vi "Setup Multiple Statistics Measurement.vi"(6 "Measurements":T1[](array[typedef]), 8 "error in (no error)":errorcluster, 10 "Channels":T2, 11 "MSOX6004 in":refnum<class "MSOX6004.lvclass">) -> (0 "error out":errorcluster, 3 "MSOX6004 out":refnum<class "MSOX6004.lvclass">)   [LabVIEW 2018, in "MSOX6004.lvlib" / "MSOX6004.lvclass"]
uses:
  MSOX6004.lvclass
  PPLs/Oscilloscope/Parent/Oscilloscope.lvlibp/Custom Controls/Analog Channels.ctl
  PPLs/Oscilloscope/Parent/Oscilloscope.lvlibp/Custom Controls/Measurement.ctl
  MSOX6004.lvclass/MSOX6004.ctl
  <instrlib>/Keysight InfiniiVision/Keysight InfiniiVision.lvlib
  PPLs/Oscilloscope/Parent/Oscilloscope.lvlibp/Oscilloscope.lvclass
  C:/Projects/LabVIEW/PPLs/Oscilloscope/Parent/Oscilloscope.lvlibp/Oscilloscope.lvclass
  PPLs/Oscilloscope/Parent/Oscilloscope.lvlibp
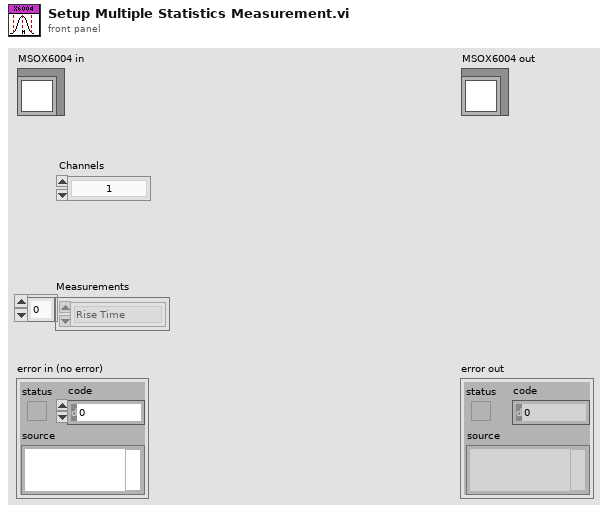
[diagram p1: front panel]
types:
  T1 = typedef "Oscilloscope.lvlibp/Measurement.ctl" = enum16{"Rise Time", "Fall Time", "Frequency", "Period", "RMS (V)", "Peak-Peak (V)", "Max (V)", "Min (V)", "High State (V)", "Low State (V)", "Average (V)", "Width (Negative)", "Width (Positive)", "Duty Cycle (Negative)", "Duty Cycle (Positive)", "Amplitude", "Cycle RMS (V)", "Cycle Avg (V)", "Overshoot", "Preshoot", "Time at Max", "Frequency Counter", "Time at Min", "Delay", "Value at Time", "Phase", "Time at Value", "Time of Edge", "Area", "Burst Width", "Falling Edge Count", "Rising Edge Count", "Falling Pulse Count", "Rising Pulse Count", "Std Dev", "Pulse Width"}
  T2 = typedef "Oscilloscope.lvlibp/Analog Channels.ctl" = enum16{"1", "2", "3", "4", "5", "6", "7", "8", "9", "10", "11", "12", "13", "14", "15", "16"}
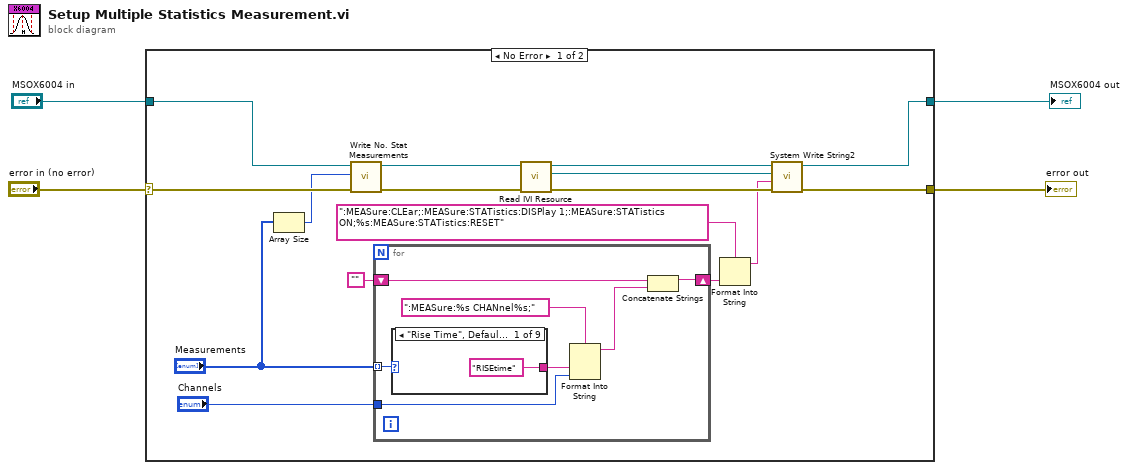
[diagram p0: block diagram]
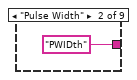
[diagram p2: hidden frame]
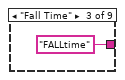
[diagram p3: hidden frame]
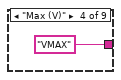
[diagram p4: hidden frame]
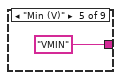
[diagram p5: hidden frame]
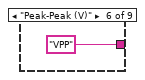
[diagram p6: hidden frame]
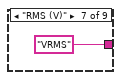
[diagram p7: hidden frame]
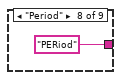
[diagram p8: hidden frame]
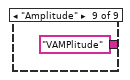
[diagram p9: hidden frame]
diagram:
  n1 = case shown="No Error" "error in (no error)" {
    selector: "error in (no error)" -> [w8 w36]
    tunnel: "MSOX6004 in" -> [w10 w37]
    tunnel: [w11 w37] -> w1
    tunnel: [w13 w36] -> w3
    frame No Error {
      n2 = Array Size(array="Measurements") -> (size(s)=w5:i32)
      n3 = call "Write No. Stat Measurements.vi"("error in (no error)"=w8, "No. Stat Measurements"=w5, "Oscilloscope in"=w10) -> ("error out"=w7:errorcluster, "Oscilloscope out"=w9:refnum<class "MSOX6004.lvclass">)  [unwired: 7 in]
      n4 = for {
        tunnel: "Measurements" -> [w26] mode=indexing
        tunnel: "Channels" -> [w24]
        shift-right: [w22] -> w17
        shift-left: "" -> [w21]
        n5 = case shown="\"Rise Time\", Default" w26 {
          tunnel: ["RISEtime" "PWIDth" "FALLtime" "VMAX" "VMIN" "VPP" "VRMS" "PERiod" "VAMPlitude"] -> w25
          frame "Rise Time", Default {
          }
          frame "Pulse Width" {
          }
          frame "Fall Time" {
          }
          frame "Max (V)" {
          }
          frame "Min (V)" {
          }
          frame "Peak-Peak (V)" {
          }
          frame "RMS (V)" {
          }
          frame "Period" {
          }
          frame "Amplitude" {
          }
        }
        n6 = Format Into String(format string=":MEASure:%s CHANnel%s;", w25, w24) -> (resulting string=w20:string)  [unwired: 2 in, 1 out]
        n7 = Concatenate Strings(w21, w20) -> (w22:string)
      }
      n8 = call "Read IVI Resource.vi"("error in (no error)"=w7, "MSOX6004 in"=w9) -> ("error out"=w15:errorcluster, "IVI Resource"=w16:refnum<k15>, "MSOX6004 out"=w11:refnum<class "MSOX6004.lvclass">)  [unwired: 7 in]
      n9 = Format Into String(format string=":MEASure:CLEar;:MEASure:STATistics:DISPlay 1;:MEASure:STATistics ON;%s:MEASure:STATistics:RESET", w17) -> (resulting string=w14:string)  [unwired: 2 in, 1 out]
      n10 = call <instrlib>:"System Write String2.vi"("error in (no error)"=w15, "Data"=w14, "instrument handle"=w16) -> ("error out"=w13:errorcluster)  [unwired: 7 in, 1 out]
    }
    frame Error {
    }
  }
  "error out" <- w3
  "MSOX6004 out" <- w1
